vi "test Read Default TagDistanceArray.vi"(8 "error in (no error)":errorcluster, 11 "TestCase in":refnum<class "AnchorTests.lvclass">) -> (0 "error out":errorcluster, 3 "TestCase out":refnum<class "AnchorTests.lvclass">)   [LabVIEW 2014, in "AnchorTests.lvclass"]
uses:
  AnchorTests.lvclass
  SPLAT/Tag.lvclass
  SPLAT/Anchor/Anchor.lvclass
  <vilib>/addons/_JKI Toolkits/VI Tester/TestCase.llb/TestCase.lvclass
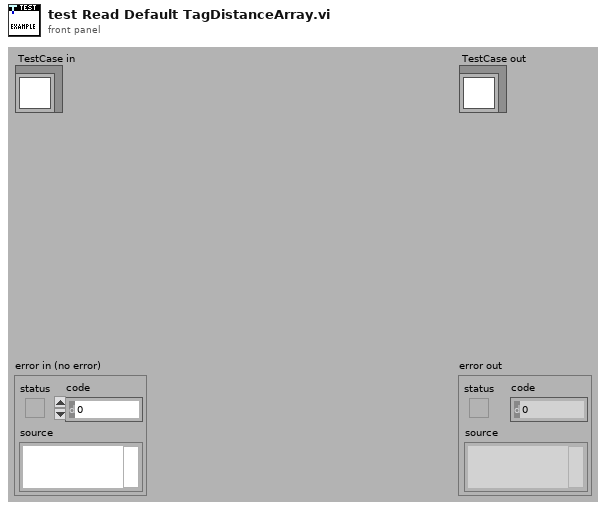
[diagram p1: front panel]
types:
  T1 = cluster{"Tag.lvclass":refnum<class "Tag.lvclass">, "Distance":dbl}[]
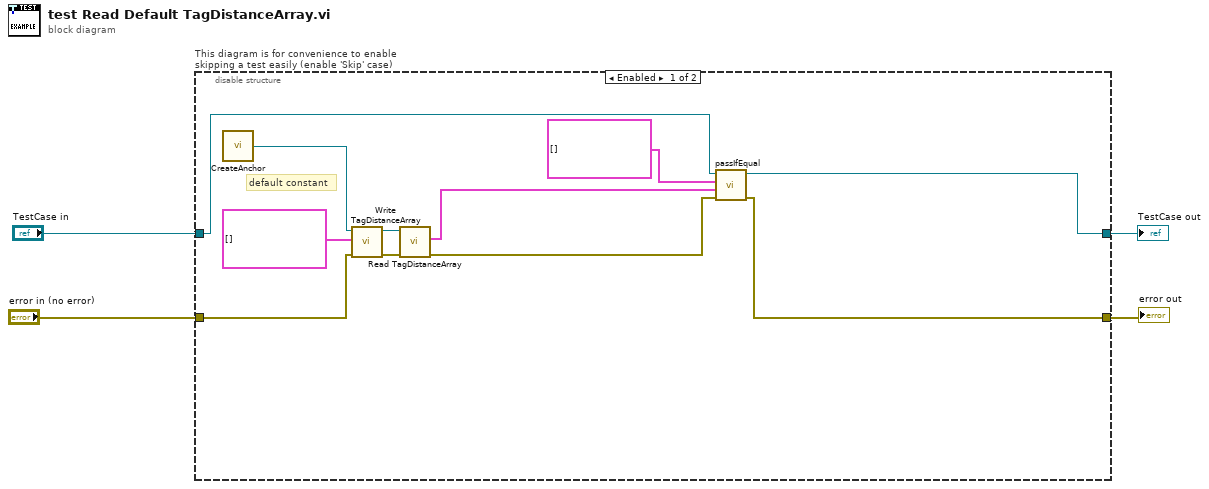
[diagram p0: block diagram]
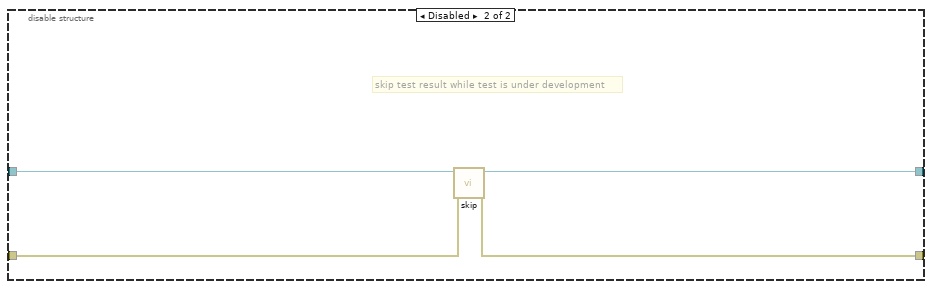
[diagram p2: hidden frame]
diagram:
  n1 = disable-structure "This diagram is for convenience to enable skipping a test easily (enable 'Skip' case)" shown="Enabled" {
    disable-tunnel: "TestCase in" -> [w7 w19]
    disable-tunnel: [w6 w17] -> w1
    disable-tunnel: [w5 w18] -> w3
    disable-tunnel: "error in (no error)" -> [w12 w16]
    frame Enabled {
      # "default constant"
      n2 = call "CreateAnchor.vi"() -> ("Anchor Out"=w14:refnum<class "Anchor.lvclass">)  [unwired: 3 in]
      n3 = call-dynamic "Write TagDistanceArray.vi"("error in (no error)"=w12, "TagDistanceArray"=T1 [], "Anchor in"=w14) -> ("error out"=w11:errorcluster, "Anchor out"=w13:refnum<class "Anchor.lvclass">)  [unwired: 7 in]
      n4 = call-dynamic "Read TagDistanceArray.vi"("error in (no error)"=w11, "Anchor in"=w13) -> ("error out"=w10:errorcluster, "TagDistanceArray"=w9:T1)  [unwired: 7 in, 1 out]
      n5 = call-dynamic "passIfEqual.vi"("error in (no error)"=w10, "y"=w9, "x"=T1 [] ("TagDistanceArray"), "TestCase in"=w7) -> ("error out"=w5:errorcluster, "TestCase out"=w6:refnum<class "AnchorTests.lvclass">)  [unwired: 6 in]
    }
    frame Disabled {
      # "skip test result while test is under development"
      n6 = call <vilib>:"skip.vi"("error in (no error)"=w16, "TestCase in"=w19) -> ("error out"=w18:errorcluster, "TestCase out"=w17:refnum<class "AnchorTests.lvclass">)  [unwired: 8 in]
    }
  }
  "error out" <- w3
  "TestCase out" <- w1
